vi "GT Active Scheduler wSubset4Tardiness.vi"(7 "Lambda":dbl, 8 "error in (no error)":errorcluster, 9 "Operation Selection Rule":T1=enum."SPT", 10 "Schedule In":u16[](array[numeric])=[12, 0, 7, 2, 6, 3, 13, 5, 1, 4, 14, 11, 10, 15, 8, 9], 11 "OSSP_Problem.lvclass":refnum<class "OSSP_Problem.lvclass">) -> (0 "error out":errorcluster, 1 "Job Completion Times":u16[](array[numeric]), 2 "Ordered Schedule Out":u16[](array[numeric]), 3 "OSSP_Problem out":refnum<class "OSSP_Problem.lvclass">, 4 "Completion Times":u16[][](array[numeric]), 5 "Start Times":u16[][](array[numeric]))   [LabVIEW 2013, in "Scheduler.lvclass"]
uses:
  Scheduler.lvclass
  OSSP_Problem.lvclass
  Operation Selection Rule from Subset to Schedule.ctl
  OSSP_Problem.lvclass/OSSP_Problem.ctl
panel:
  out "Machine Completion Times":u16[](array[numeric])
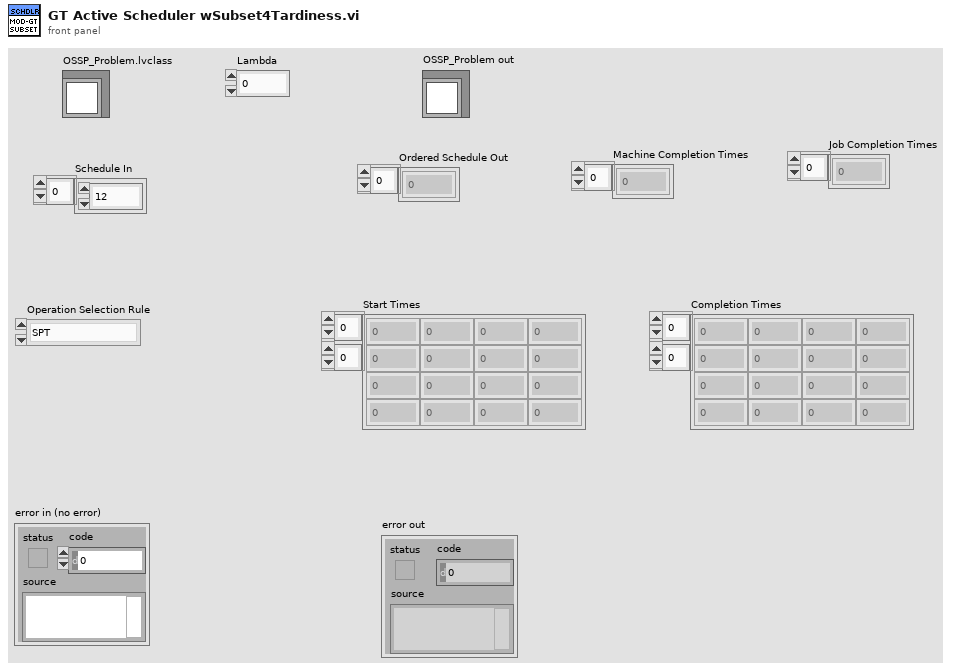
[diagram p1: front panel]
types:
  T1 = typedef "Scheduler.lvclass/Operation Selection Rule from Subset to Schedule.ctl" = enum16{"First Operation in Order", "SPT", "EDD", "MDD"}
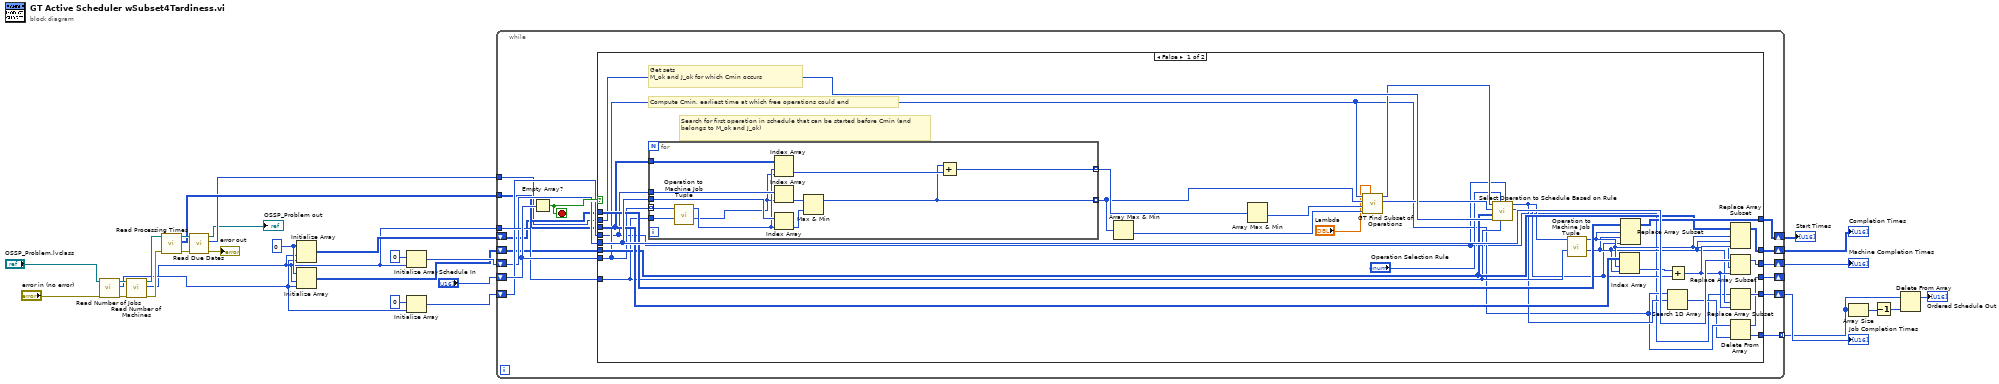
[diagram p0: block diagram]
diagram:
  w23 = u16 0 ("element")
  n1 = call "Read Number of Jobs.vi"("error in (no error)"="error in (no error)", "OSSP_Problem in"="OSSP_Problem.lvclass") -> ("error out"=w9:errorcluster, "Number of Jobs"=w6:i32, "OSSP_Problem out"=w13:refnum<class "OSSP_Problem.lvclass">)  [unwired: 7 in]
  n2 = call "Read Number of Machines.vi"("error in (no error)"=w9, "OSSP_Problem in"=w13) -> ("error out"=w8:errorcluster, "Number of Machines"=w5:i32, "OSSP_Problem out"=w12:refnum<class "OSSP_Problem.lvclass">)  [unwired: 7 in]
  n3 = call "Read Processing Times.vi"("error in (no error)"=w8, "OSSP_Problem in"=w12) -> ("error out"=w7:errorcluster, "Processing Times"=w4:u16[][], "OSSP_Problem out"=w11:refnum<class "OSSP_Problem.lvclass">)  [unwired: 7 in]
  n4 = call "Read Due Dates.vi"("error in (no error)"=w7, "OSSP_Problem in"=w11) -> ("error out"=→"error out":errorcluster, "Due Dates"=w3:u16[], "OSSP_Problem out"=→"OSSP_Problem out":refnum<class "OSSP_Problem.lvclass">)  [unwired: 7 in]
  n5 = Initialize Array(w23, w5, w6) -> (w22:u16[][])
  n6 = Initialize Array(w23, w5, w6) -> (w15:u16[][])
  n7 = Initialize Array(u16 0 ("element"), w5) -> (w27:u16[])
  n8 = Initialize Array(u16 0 ("element"), w6) -> (w28:u16[])
  n9 = while {
    shift-right: [w37] -> _
    shift-left: "Schedule In" -> [w44]
    tunnel: w5 -> [w43]
    shift-right: [w40] -> w26
    shift-left: w28 -> [w42]
    shift-right: [w39] -> w25
    shift-left: w27 -> [w41]
    shift-right: [w35] -> w16
    shift-left: w15 -> [w36]
    tunnel: w4 -> [w38]
    shift-right: [w33] -> w17
    shift-left: w22 -> [w34]
    tunnel: [w32] -> w18 mode=indexing
    tunnel: w3 -> [w31]
    stop <- w45 stop-if-true
    n10 = Empty Array?(array=w44) -> (empty?=w45:bool)
    n11 = case shown="False" w45 {
      tunnel: w44 -> [w51 w89]
      tunnel: w43 -> [w57 _]
      tunnel: w42 -> [w46 w91]
      tunnel: w41 -> [w74 w90]
      tunnel: [w73 w91] -> w40
      tunnel: [w72 w90] -> w39
      tunnel: w38 -> [w63 _]
      tunnel: [w66 w89] -> w37
      tunnel: w36 -> [w61 w88]
      tunnel: [w71 w88] -> w35
      tunnel: w34 -> [w70 w87]
      tunnel: [w69 w87] -> w33
      tunnel: [w65 _] -> w32
      tunnel: w31 -> [w62 _]
      frame False {
        # "Search for first operation in schedule that can be started before Cmin (and belongs to M_ok and J_ok)"
        # "Get sets \nM_ok and J_ok for which Cmin occurs"
        # "Compute Cmin, earliest time at which free operations could end"
        n12 = for {
          tunnel: w51 -> [w86] mode=indexing
          tunnel: w57 -> [w85]
          tunnel: w46 -> [w83]
          tunnel: w74 -> [w84]
          tunnel: [w76] -> w68 mode=indexing
          tunnel: w63 -> [w80]
          tunnel: [w75] -> w49 mode=indexing
          n13 = call "Operation to Machine Job Tuple.vi"("Number of Machines"=w85, "Operation Number"=w86) -> ("Job No"=w78:i32, "Machine No"=w79:i32)  [unwired: 8 in]
          n14 = Index Array(array=w80, index (row)=w79, index (col)=w78) -> (element=w77:u16)
          n15 = Index Array(array=w83, index=w78) -> (element=w82:u16)
          n16 = Index Array(array=w84, index=w79) -> (element=w81:u16)
          n17 = Max & Min(x=w82, y=w81) -> (max(x,y)=w75:u16)  [unwired: 1 out]
          n18 = Add(x=w75, y=w77) -> (x+y=w76:u16)
        }
        n19 = Array Max & Min(array=w49) -> (min value=w48:u16)  [unwired: 3 out]
        n20 = Array Max & Min(array=w68) -> (min value=w64:u16)  [unwired: 3 out]
        n21 = call "GT Find Subset of Operations.vi"("Lambda"="Lambda", "ESmin"=w48, "ECmin"=w64, "Earliest Start Times Array"=w49, "Schedule"=w51) -> ("ES Times  SubSet Out"=w60:u16[], "Operation  Subset Out"=w59:u16[])  [unwired: 5 in]
        n22 = call "Select Operation to Schedule Based on Rule.vi"("EOJ"=w46, "Number of Machines"=w57, "Operation Selection Rule"="Operation Selection Rule", "Due Dates"=w62, "Processing Times"=w61, "ES Subset"=w60, "Operation Subset"=w59) -> ("Selected Operation's Start Time"=w53:u16, "Selected Operation for Scheduling"=w52:u16)  [unwired: 3 in]
        n23 = call "Operation to Machine Job Tuple.vi"("Number of Machines"=w57, "Operation Number"=w52) -> ("Job No"=w54:i32, "Machine No"=w55:i32)  [unwired: 8 in]
        n24 = Index Array(array=w63, index (row)=w55, index (col)=w54) -> (element=w67:u16)
        n25 = Replace Array Subset(array=w70, new element=w53, index (row)=w55, index (col)=w54) -> (w69:u16[][])
        n26 = Search 1D Array(1D array=w51, element=w52) -> (index of element=w50:i32)  [unwired: 1 in]
        n27 = Add(x=w67, y=w53) -> (x+y=w56:u16)
        n28 = Replace Array Subset(array=w61, new element=w56, index (row)=w55, index (col)=w54) -> (w71:u16[][])
        n29 = Replace Array Subset(array=w74, new element=w56, index=w55) -> (w72:u16[])
        n30 = Replace Array Subset(array=w46, new element=w56, index=w54) -> (w73:u16[])
        n31 = Delete From Array(array=w51, index=w50) -> (deleted portion=w65:u16, array with subset deleted=w66:u16[])  [unwired: 1 in]
      }
      frame True {
      }
    }
  }
  "Completion Times" <- w16
  "Job Completion Times" <- w26
  "Machine Completion Times" <- w25
  "Start Times" <- w17
  n32 = Array Size(array=w18) -> (size(s)=w21:i32)
  n33 = Decrement(x=w21) -> (x-1=w20:i32)
  n34 = Delete From Array(array=w18, index=w20) -> (array with subset deleted=→"Ordered Schedule Out":u16[])  [unwired: 1 in, 1 out]
